vi "WaterToday.vi"(10 "Day of week":i32, 11 "Cluster":T1 {"Liter" min=0.0; "Set Time" format="%<%H:%M:%S>t"; "Duration[S]" min=0.0}) -> (3 "WaterToday":bool)   [LabVIEW 2021, in "TimeBasedProd.lvlib"]
uses:
  TimeBasedProd.lvlib
  TypeDef/Time_Table_CTR.ctl
panel:
  # "Watering Days"
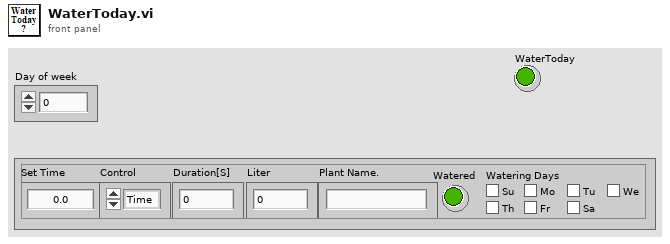
[diagram p1: front panel]
types:
  T1 = typedef "TimeBasedProd.lvlib/Time_Table_CTR.ctl" = cluster{"Set Time":dbl, "Control":enum16{"Time", "Flow"}, "Duration[S]":dbl, "Liter":dbl, "Plant Name.":string, "Watered":bool, "Su":bool, "Mo":bool, "Tu":bool, "We":bool, "Th":bool, "Fr":bool, "Sa":bool}
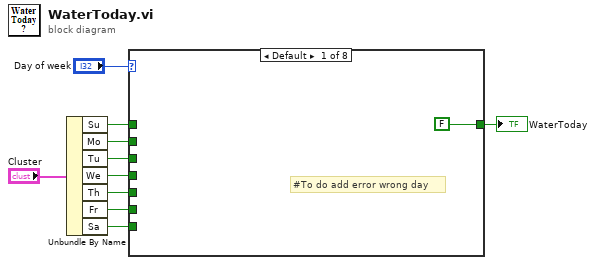
[diagram p0: block diagram]
diagram:
  n1 = Unbundle By Name("Cluster") -> ("Su"=w9:bool, "Mo"=w8:bool, "Tu"=w7:bool, "We"=w6:bool, "Th"=w5:bool, "Fr"=w4:bool, "Sa"=w3:bool)
  n2 = case shown="Default" "Day of week" {
    tunnel: [FALSE ("Sa") w12 w13 w14 w15 w16 w17 w18] -> w1
    tunnel: w9 -> [_ w12 _ _ _ _ _ _]
    tunnel: w8 -> [_ _ w13 _ _ _ _ _]
    tunnel: w7 -> [_ _ _ w14 _ _ _ _]
    tunnel: w6 -> [_ _ _ _ w15 _ _ _]
    tunnel: w5 -> [_ _ _ _ _ w16 _ _]
    tunnel: w4 -> [_ _ _ _ _ _ w17 _]
    tunnel: w3 -> [_ _ _ _ _ _ _ w18]
    frame Default {
      # "#To do add error wrong day"
    }
    frame 0 {
    }
    frame 1 {
    }
    frame 2 {
    }
    frame 3 {
    }
    frame 4 {
    }
    frame 5 {
    }
    frame 6 {
    }
  }
  "WaterToday" <- w1
